vi "calculator.vi"() -> ()   [LabVIEW 2016]
uses:
  Control 1.ctl
panel:
  out "used time":T1
  out "now time":timestamp
  out "Boolean 34":bool
  out "Boolean 33":bool
  out "Boolean 32":bool
  out "Boolean 31":bool
  out "Boolean 30":bool
  in  "）":bool
  in  "（":bool
  in  "Lock Button":bool
  in  "Clear":bool
  in  "Allclear":bool
  out "Boolean 27":bool
  out "Boolean 26":bool
  out "Boolean 25":bool
  out "Boolean 24":bool
  out "Boolean 23":bool
  out "Boolean 22":bool
  out "Boolean 21":bool
  out "Boolean 20":bool
  in  "stored":dbl format="%#_15f"
  out "Boolean 19":bool
  out "Boolean 18":bool
  out "Boolean 17":bool
  out "Boolean 16":bool
  out "Boolean 15":bool
  out "Boolean 14":bool
  out "Boolean 13":bool
  out "Boolean 12":bool
  out "Boolean 11":bool
  out "Boolean 10":bool
  in  "stop 2":bool
  out "Boolean 9":bool
  out "Boolean 8":bool
  out "Boolean 7":bool
  out "Boolean 6":bool
  out "Boolean 5":bool
  out "Boolean 4":bool
  out "Boolean 3":bool
  out "Boolean":bool
  out "Boolean 2":bool
  out "Boolean":bool
  in  "exp":bool
  in  "reciprocal":bool
  in  "cube":bool
  in  "cosine":bool
  in  "sine":bool
  in  "tangent":bool
  in  "+-":bool
  in  "root":bool
  in  "square":bool
  in  "+":bool
  in  "*":bool
  in  "-":bool
  in  "/":bool
  in  "3":bool
  in  "stop":bool
  in  "顯示":dbl format="%#_15f"
  in  "0":bool
  in  ".":bool
  in  "9":bool
  in  "8":bool
  in  "7":bool
  in  "6":bool
  in  "5":bool
  in  "4":bool
  in  "2":bool
  in  "=":bool
  in  "1":bool
  # "stored"
  # "now"
  # "parameter lock"
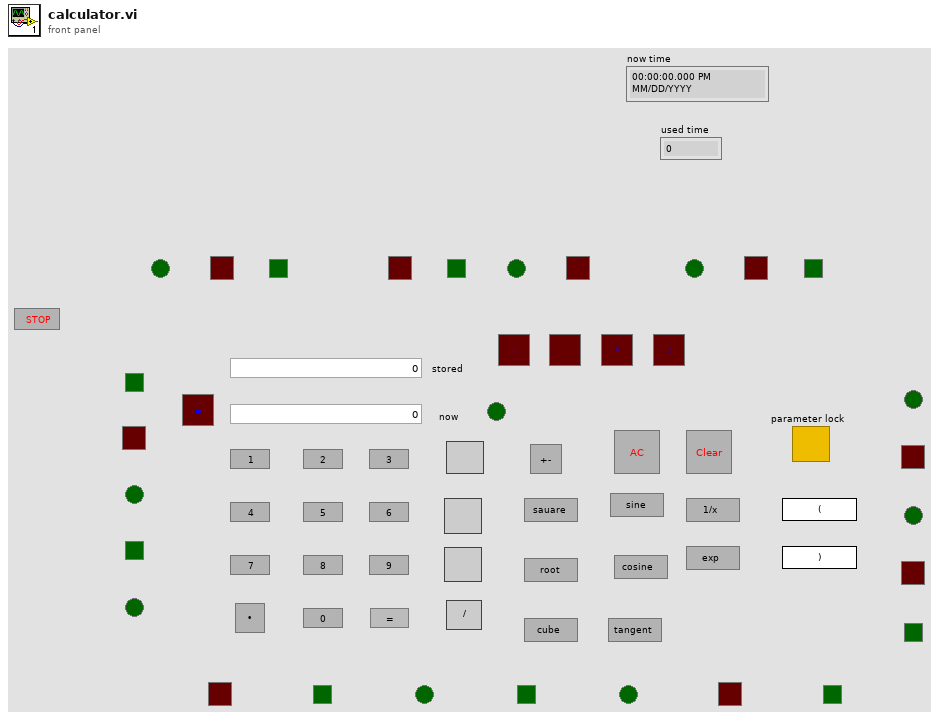
[diagram p1: front panel]
types:
  T1 = typedef "Control 1.ctl" = dbl
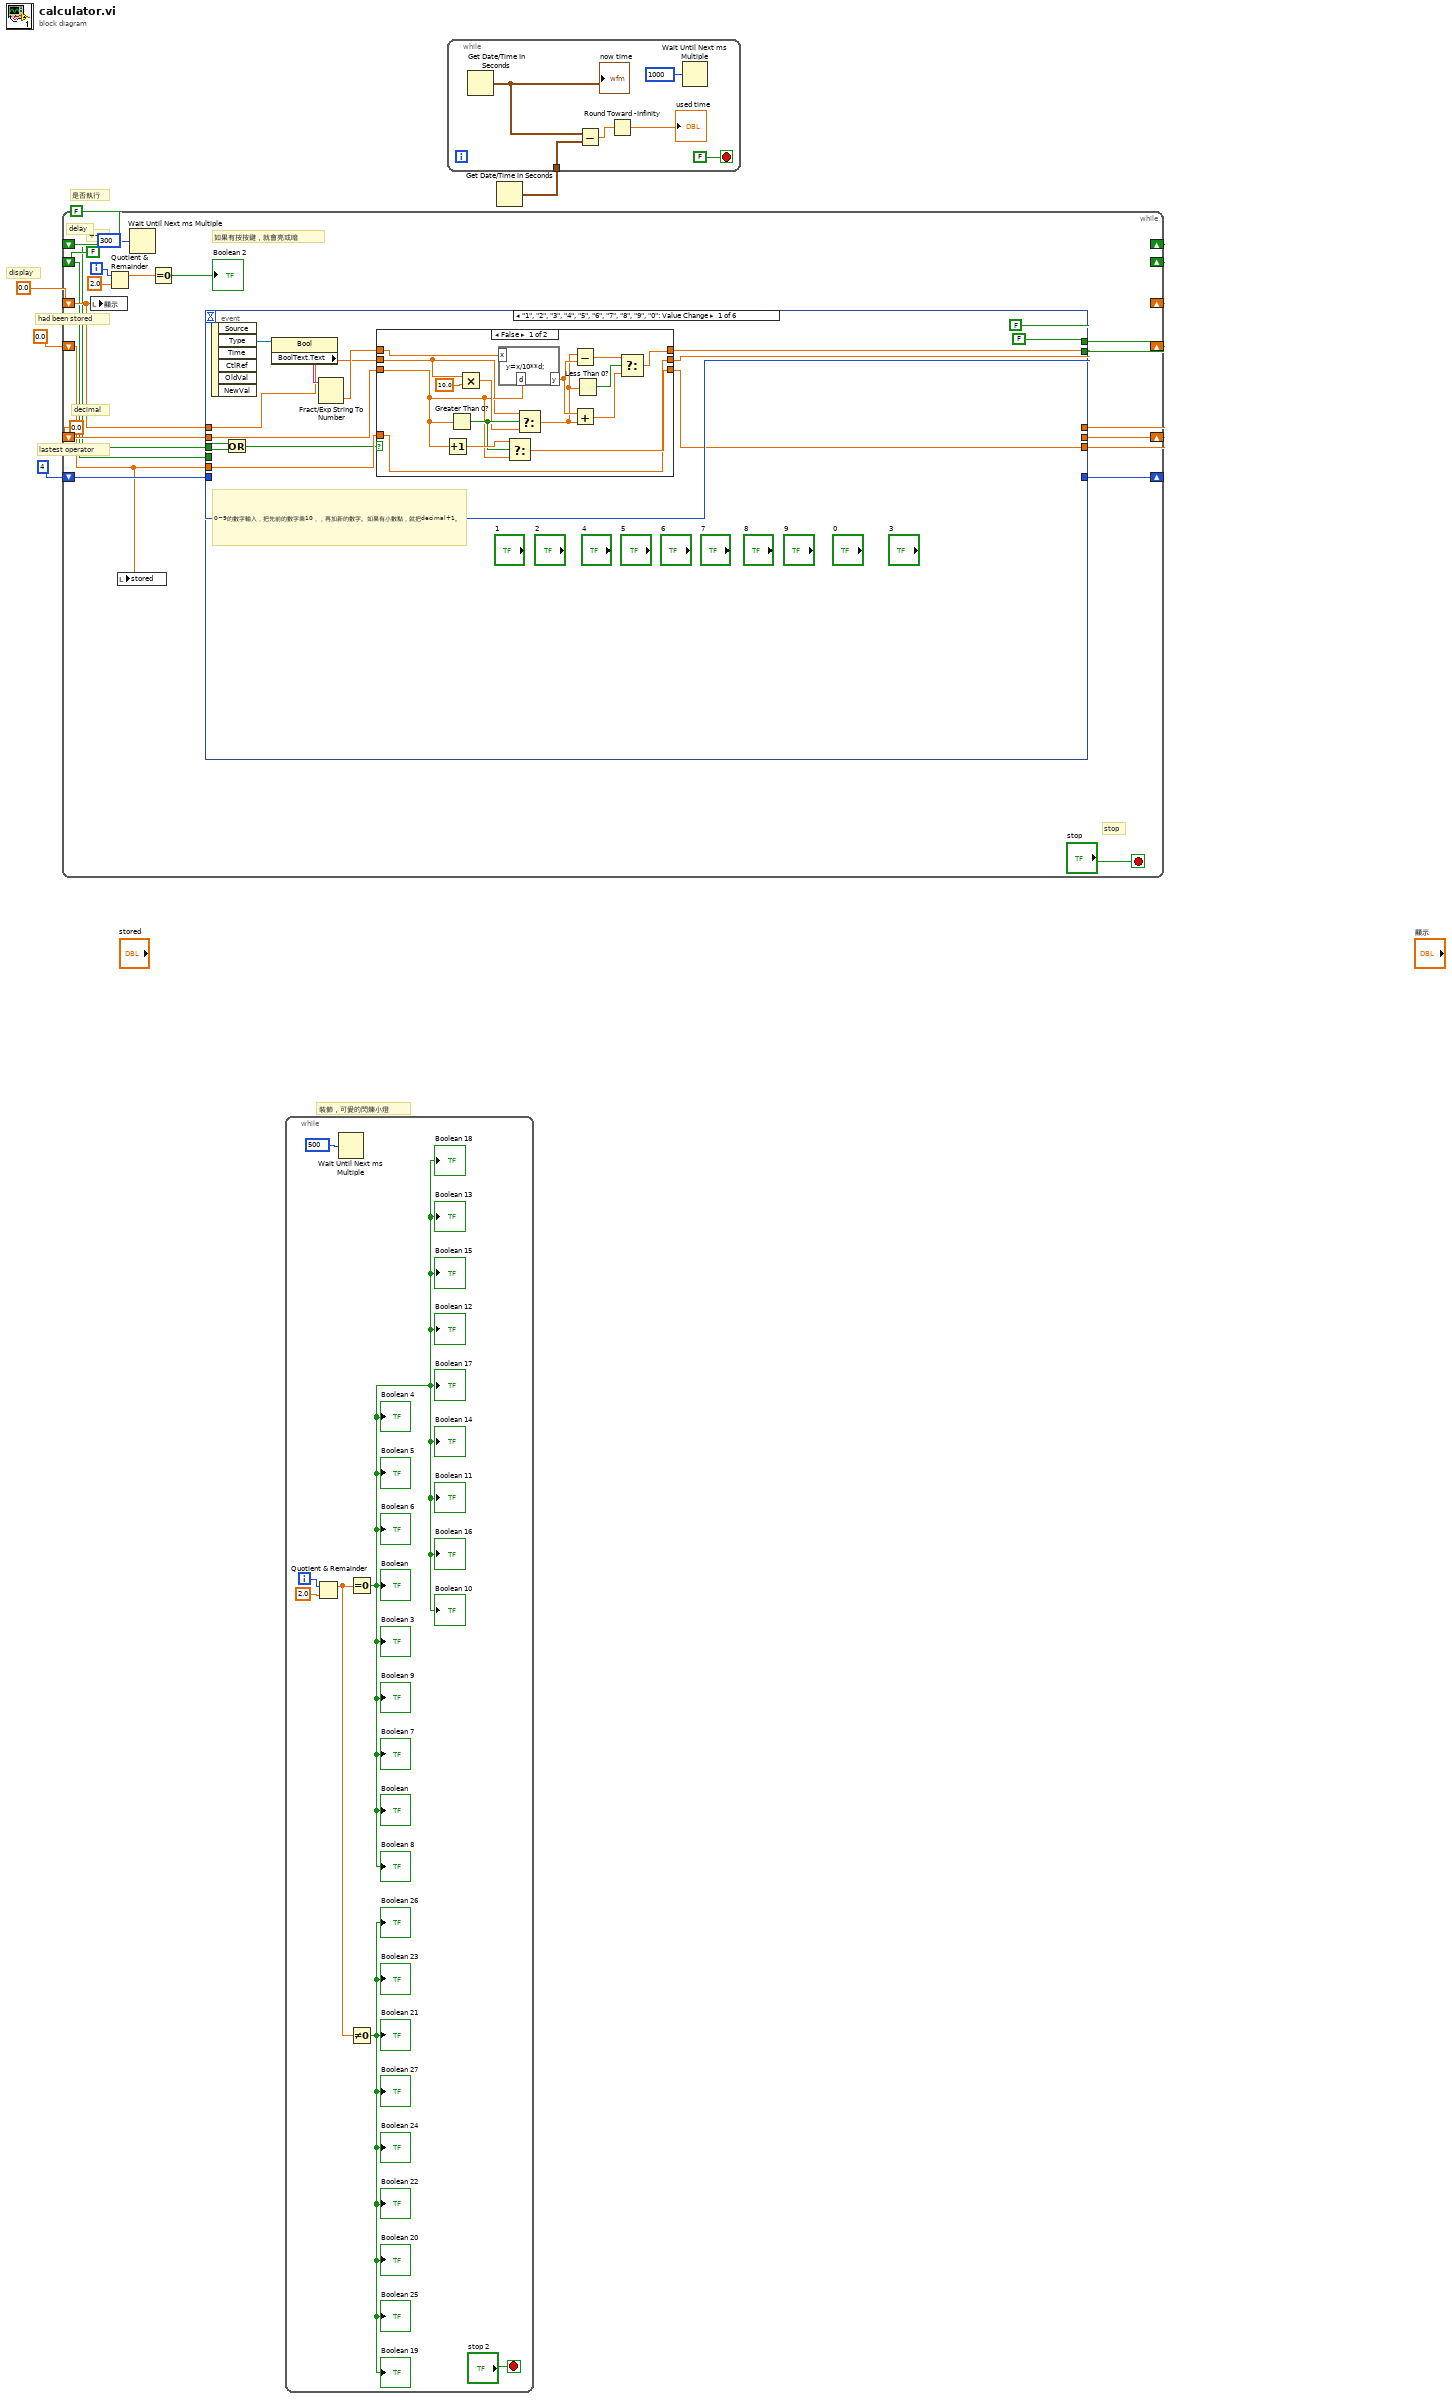
[diagram p0: block diagram]
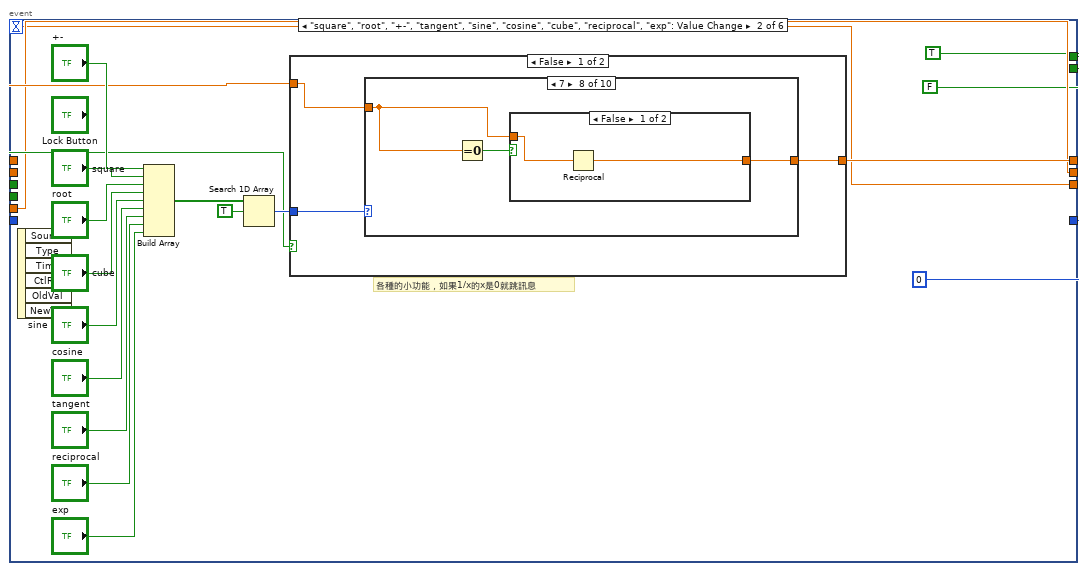
[diagram p3: hidden frame]
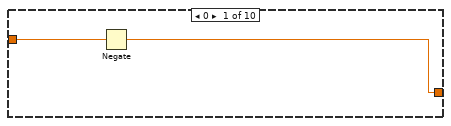
[diagram p4: hidden frame]
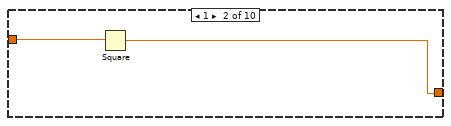
[diagram p5: hidden frame]
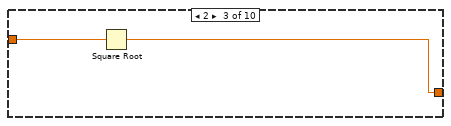
[diagram p6: hidden frame]
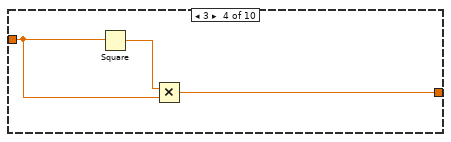
[diagram p7: hidden frame]
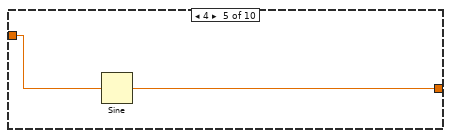
[diagram p8: hidden frame]
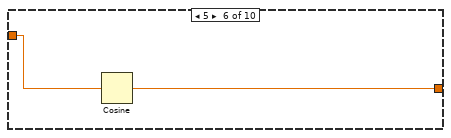
[diagram p9: hidden frame]
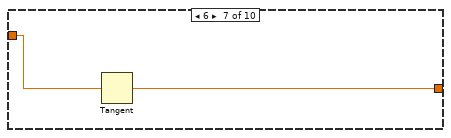
[diagram p10: hidden frame]
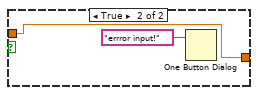
[diagram p11: hidden frame]
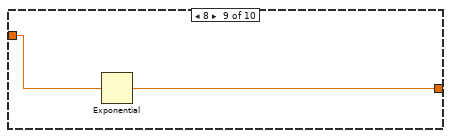
[diagram p12: hidden frame]
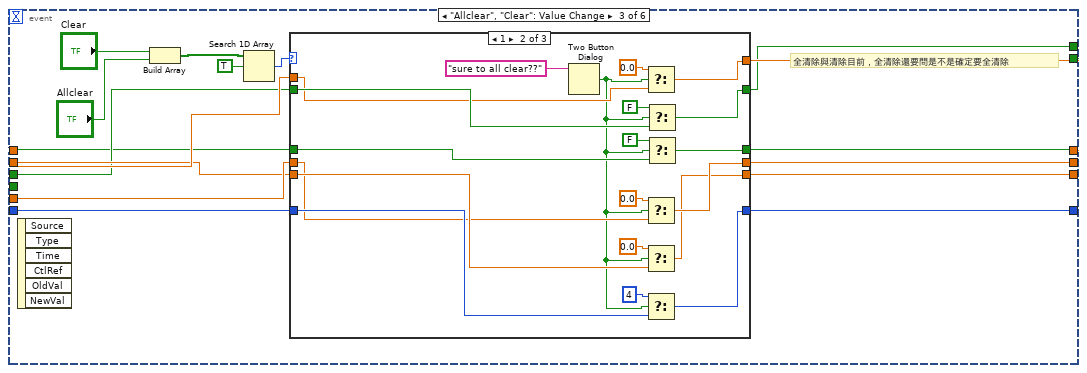
[diagram p15: hidden frame]
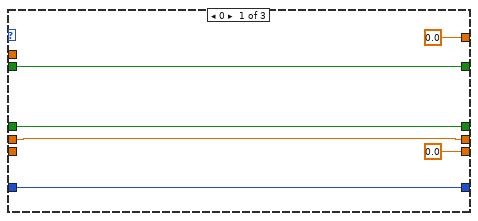
[diagram p16: hidden frame]
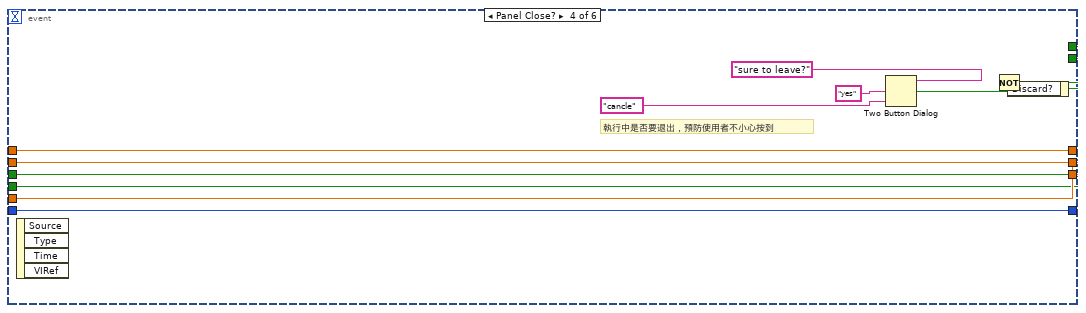
[diagram p18: hidden frame]
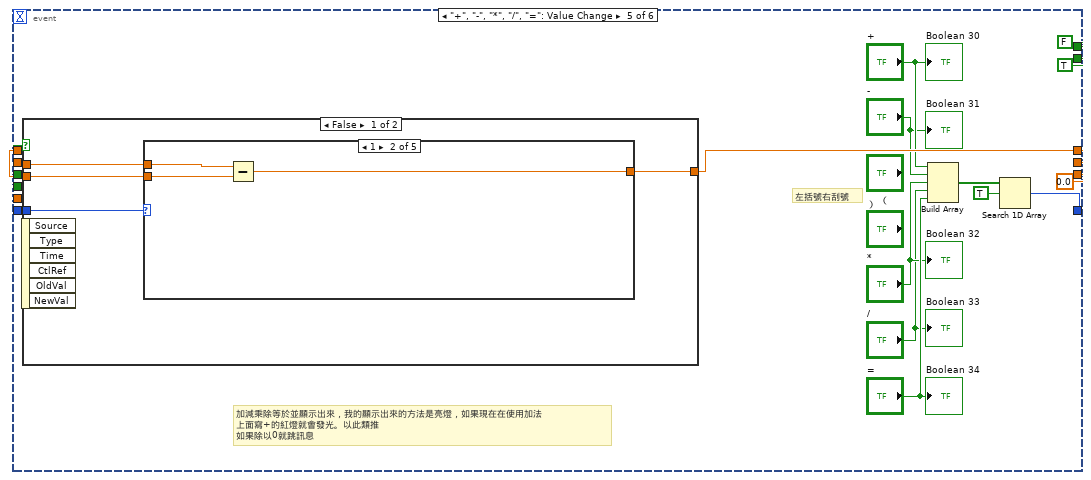
[diagram p19: hidden frame]
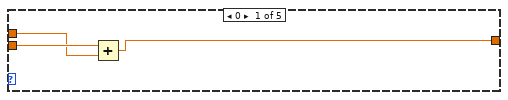
[diagram p20: hidden frame]
diagram:
  # "是否執行"
  # "裝飾，可愛的閃爍小燈"
  # "+-*/"
  # "had been stored"
  # "lastest operator"
  # "display"
  # "decimal"
  n1 = while {
    shift-right: [w23] -> _
    shift-left: 0.0 ("Numeric") -> [w24]
    shift-right: [w22] -> _
    shift-left: 0.0 ("Numeric") -> [w21]
    shift-right: [w20] -> _
    shift-left: 4 -> [w19]
    shift-right: [w18] -> _
    shift-left: 0.0 -> [w8]
    shift-right: [w17] -> _
    shift-left: FALSE -> [w16]
    shift-right: [w10] -> _
    shift-left: FALSE -> [w9]
    i -> [w11]
    stop <- "stop" stop-if-true
    # "stop"
    # "如果有按按鍵，就會亮或暗"
    # "delay"
    n2 = local write "顯示"(w24) -> ()
    n3 = Quotient & Remainder(x=w11, y=2.0) -> (x-y*floor(x/y)=w13:dbl)  [unwired: 1 out]
    n4 = local write "stored"(w8) -> ()
    n5 = Wait Until Next ms Multiple(millisecond multiple=u32 300) -> ()  [unwired: 1 out]
    n6 = Equal To 0?(x=w13) -> (x = 0?=→"Boolean 2":bool)
    n7 = event shown="[0] \"1\", \"2\", \"3\", \"4\", \"5\", \"6\", \"7\", \"8\", \"9\", \"0\": Value Change" {
      selector: _ -> [_ _ _ _ _ _]
      dyn-events: _ -> [_ _ _ _ _ _]
      timeout: _ -> [_ _ _ _ _ _]
      tunnel: w24 -> [w34 w72 w120 w164 w180 w215]
      tunnel: [w32 w71 w115 w164 w179 w215] -> w23
      tunnel: [w33 w59 w113 w162 0.0 w210] -> w22
      tunnel: w21 -> [w36 w59 w118 w162 _ w211]
      tunnel: [w38 0 ("index of element") w112 w161 w176 w214] -> w20
      tunnel: w19 -> [w38 _ w117 w161 w181 w214]
      tunnel: [w30 w68 w114 w163 w179 w208] -> w18
      tunnel: [FALSE FALSE w111 w160 TRUE FALSE] -> w17
      tunnel: w16 -> [w29 w70 w108 w160 w174 _]
      tunnel: w8 -> [w31 w68 w119 w163 w175 w208]
      tunnel: w9 -> [w28 _ w116 w159 _ _]
      tunnel: [FALSE TRUE w110 w159 FALSE _] -> w10
      event "1", "2", "3", "4", "5", "6", "7", "8", "9", "0": Value Change {
        # "0~9的數字輸入，把先前的數字乘10，，再加新的數字。如果有小數點，就把decimal+1。"
        n8 = event-data() -> ("CtlRef"=w39:refnum<vi>)  [unwired: 1 in, 5 out]
        n9 = Or(x=w29, y=w28) -> (x .or. y?=w27:bool)
        n10 = property class="Bool"(reference=w39) -> ("BoolText.Text"=w40:string)  [unwired: 1 in, 2 out]
        n11 = Fract/Exp String To Number(string=w40) -> (number=w35:dbl)  [unwired: 3 in, 1 out]
        n12 = case shown="False" w27 {
          tunnel: w36 -> [w43 w58]
          tunnel: [w46 w57] -> w32
          tunnel: [w45 w58] -> w33
          tunnel: w35 -> [w44 w57]
          tunnel: w34 -> [w41 w56]
          tunnel: w31 -> [w42 _]
          tunnel: [w42 w56] -> w30
          frame False {
            n13 = Increment(x=w43) -> (x+1=w55:dbl)
            n14 = Greater Than 0?(x=w43) -> (x > 0?=w54:bool)
            n15 = Multiply(x=w41, y=10.0 ("Numeric")) -> (x*y=w52:dbl)
            n16 = formula code="y=x/10**d;"("x"=w44, "d"=w43) -> ("y"=w53:dbl)
            n17 = Select(t=w55, s=w54, f=w43) -> (s? t:f=w45:dbl)
            n18 = Select(t=w41, s=w54, f=w52) -> (s? t:f=w51:dbl)
            n19 = Subtract(x=w51, y=w53) -> (x-y=w49:dbl)
            n20 = Add(x=w53, y=w51) -> (x+y=w50:dbl)
            n21 = Less Than 0?(x=w51) -> (x < 0?=w48:bool)
            n22 = Select(t=w49, s=w48, f=w50) -> (s? t:f=w46:dbl)
          }
          frame True {
          }
        }
      }
      event "square", "root", "+-", "tangent", "sine", "cosine", "cube", "reciprocal", "exp": Value Change {
        # "各種的小功能，如果1/x的x是0就跳訊息"
        n23 = event-data() -> ()  [unwired: 1 in, 6 out]
        n24 = Build Array("+-", "square", "root", "cube", "sine", "cosine", "tangent", "reciprocal", "exp") -> (w74:bool[])
        n25 = Search 1D Array(1D array=w74, element=TRUE) -> (index of element=w73:i32)  [unwired: 1 in]
        n26 = case shown="False" w70 {
          tunnel: w73 -> [w81 _]
          tunnel: w72 -> [w80 w107]
          tunnel: [w79 w107] -> w71
          frame False {
            n27 = case shown="7" w81 {
              tunnel: w80 -> [w83 w85 w87 w88 w92 w94 w96 w98 w105 w106]
              tunnel: [w82 w84 w86 w89 w91 w93 w95 w97 w104 w106] -> w79
              frame 0 {
                n28 = Negate(x=w83) -> (-x=w82:dbl)
              }
              frame 1 {
                n29 = Square(x=w85) -> (x^2=w84:dbl)
              }
              frame 2 {
                n30 = Square Root(x=w87) -> (sqrt(x)=w86:dbl)
              }
              frame 3 {
                n31 = Square(x=w88) -> (x^2=w90:dbl)
                n32 = Multiply(x=w90, y=w88) -> (x*y=w89:dbl)
              }
              frame 4 {
                n33 = Sine(x=w92) -> (sin(x)=w91:dbl)
              }
              frame 5 {
                n34 = Cosine(x=w94) -> (cos(x)=w93:dbl)
              }
              frame 6 {
                n35 = Tangent(1:w96) -> (0:w95:dbl)
              }
              frame 7 {
                n36 = Equal To 0?(x=w98) -> (x = 0?=w99:bool)
                n37 = case shown="False" w99 {
                  tunnel: [w100 w102] -> w97
                  tunnel: w98 -> [w101 w102]
                  frame False {
                    n38 = Reciprocal(x=w101) -> (1/x=w100:dbl)
                  }
                  frame True {
                    n39 = One Button Dialog(message="errror input!") -> ()  [unwired: 1 in, 1 out]
                  }
                }
              }
              frame 8 {
                n40 = Exponential(1:w105) -> (0:w104:dbl)
              }
              frame Default {
              }
            }
          }
          frame True {
          }
        }
      }
      event "Allclear", "Clear": Value Change {
        # "全清除與清除目前，全清除還要問是不是確定要全清除"
        n41 = event-data() -> ()  [unwired: 1 in, 6 out]
        n42 = Build Array("Clear", "Allclear") -> (w122:bool[])
        n43 = Search 1D Array(1D array=w122, element=TRUE) -> (index of element=w109:i32)  [unwired: 1 in]
        n44 = case shown="1" w109 {
          tunnel: w120 -> [_ w134 w156]
          tunnel: w119 -> [w130 w135 w155]
          tunnel: w118 -> [_ w136 w154]
          tunnel: w117 -> [w127 w137 w153]
          tunnel: w116 -> [w126 w139 w152]
          tunnel: [0.0 ("Numeric") w149 w156] -> w115
          tunnel: [w130 w148 w155] -> w114
          tunnel: [0.0 ("Numeric") w147 w154] -> w113
          tunnel: [w127 w146 w153] -> w112
          tunnel: [w125 w132 w151] -> w111
          tunnel: [w126 w131 w152] -> w110
          tunnel: w108 -> [w125 w138 w151]
          frame 0 {
          }
          frame 1 {
            n45 = Two Button Dialog(message="sure to all clear??") -> (T button?=w133:bool)  [unwired: 2 in]
            n46 = Select(t=0.0 ("Numeric"), s=w133, f=w134) -> (s? t:f=w149:dbl)
            n47 = Select(t=0.0, s=w133, f=w135) -> (s? t:f=w148:dbl)
            n48 = Select(t=0.0 ("Numeric"), s=w133, f=w136) -> (s? t:f=w147:dbl)
            n49 = Select(t=4, s=w133, f=w137) -> (s? t:f=w146:i32)
            n50 = Select(t=FALSE, s=w133, f=w139) -> (s? t:f=w131:bool)
            n51 = Select(t=FALSE, s=w133, f=w138) -> (s? t:f=w132:bool)
          }
          frame Default {
          }
        }
      }
      event Panel Close? {
        # "執行中是否要退出，預防使用者不小心按到"
        n52 = event-data() -> ()  [unwired: 1 in, 4 out]
        n53 = Two Button Dialog(message="sure to leave?", 1:"cancle" ("F button name (\"Cancel\")"), 2:"yes" ("T button name (\"OK\")")) -> (T button?=w158:bool)
        n54 = Not(x=w158) -> (.not. x?=w157:bool)
        n55 = event-data("Discard?"=w157) -> ()  [unwired: 1 in, 1 out]
      }
      event "+", "-", "*", "/", "=": Value Change {
        # "左括號右刮號"
        # "加減乘除等於並顯示出來，我的顯示出來的方法是亮燈，如果現在在使用加法\n上面寫+的紅燈就會發光。以此類推\n如果除以0就跳訊息"
        n56 = event-data() -> ()  [unwired: 1 in, 6 out]
        n57 = case shown="False" w174 {
          tunnel: w181 -> [w187 _]
          tunnel: w180 -> [w186 w207]
          tunnel: [w184 w207] -> w179
          tunnel: w175 -> [w185 _]
          frame False {
            n58 = case shown="1" w187 {
              tunnel: w186 -> [w190 w193 w196 w199 w206]
              tunnel: [w189 w192 w195 w197 w206] -> w184
              tunnel: w185 -> [w188 w191 w194 w198 _]
              frame 0 {
                n59 = Add(x=w190, y=w188) -> (x+y=w189:dbl)
              }
              frame 1 {
                n60 = Subtract(x=w191, y=w193) -> (x-y=w192:dbl)
              }
              frame 2 {
                n61 = Multiply(x=w194, y=w196) -> (x*y=w195:dbl)
              }
              frame 3 {
                n62 = Equal To 0?(x=w199) -> (x = 0?=w200:bool)
                n63 = case shown="True" w200 {
                  tunnel: w199 -> [w203 _]
                  tunnel: w198 -> [w202 w204]
                  tunnel: [w201 w204] -> w197
                  frame False {
                    n64 = Divide(x=w202, y=w203) -> (x/y=w201:dbl)
                  }
                  frame True {
                    n65 = One Button Dialog(message="errror input!") -> ()  [unwired: 1 in, 1 out]
                  }
                }
              }
              frame 4, Default {
              }
            }
          }
          frame True {
          }
        }
        n66 = Build Array("+", "-", "*", "/", "=") -> (w183:bool[])
        n67 = Search 1D Array(1D array=w183, element=TRUE) -> (index of element=w176:i32)  [unwired: 1 in]
        "Boolean 30" <- "+"
        "Boolean 31" <- "-"
        "Boolean 32" <- "*"
        "Boolean 33" <- "/"
        "Boolean 34" <- "="
      }
      event ".": Value Change {
        # "如果按下小數點，那decimal=1\n開始輸入小數"
        n68 = event-data() -> ()  [unwired: 1 in, 6 out]
        n69 = Equal To 0?(x=w211) -> (x = 0?=w212:bool)
        n70 = Select(t=1, s=w212, f=w211) -> (s? t:f=w210:dbl)
        n71 = Format Date/Time String() -> ()  [unwired: 3 in, 1 out]
      }
    }
  }
  n72 = while {
    i -> [w220]
    stop <- "stop 2" stop-if-true
    n73 = Quotient & Remainder(x=w220, y=2.0) -> (x-y*floor(x/y)=w218:dbl)  [unwired: 1 out]
    n74 = Wait Until Next ms Multiple(millisecond multiple=u32 500) -> ()  [unwired: 1 out]
    n75 = Equal To 0?(x=w218) -> (x = 0?=→"Boolean" →"Boolean 8" →"Boolean 9" →"Boolean 7" →"Boolean" →"Boolean 3" →"Boolean 5" →"Boolean 6" →"Boolean 18" →"Boolean 12" →"Boolean 17" →"Boolean 16" →"Boolean 10" →"Boolean 15" →"Boolean 14" →"Boolean 4" →"Boolean 13" →"Boolean 11":bool)
    n76 = Not Equal To 0?(x=w218) -> (x != 0?=→"Boolean 20" →"Boolean 24" →"Boolean 23" →"Boolean 21" →"Boolean 27" →"Boolean 26" →"Boolean 25" →"Boolean 22" →"Boolean 19":bool)
  }
  n77 = Get Date/Time In Seconds() -> (seconds since 1Jan1904=w1:timestamp)
  n78 = while {
    tunnel: w1 -> [w227]
    stop <- FALSE stop-if-true
    n79 = Get Date/Time In Seconds() -> (seconds since 1Jan1904=w226:timestamp)
    "now time" <- w226
    n80 = Subtract(x=w226, y=w227) -> (x-y=w224:dbl)
    n81 = Round Toward -Infinity(1:w224) -> (0:→"used time":dbl)
    n82 = Wait Until Next ms Multiple(millisecond multiple=u32 1000) -> ()  [unwired: 1 out]
  }
